vi "test_LogFile Exists on Windows.vi"(8 "error in (no error)":errorcluster, 11 "TestCase in":refnum<class "Telemetry System Tests.lvclass">) -> (0 "error out":errorcluster, 3 "TestCase out":refnum<class "Telemetry System Tests.lvclass">)   [LabVIEW 2019]
uses:
  Telemetry System Tests.lvclass
  e98a7768-7ae7-490c-bb08-fb750c513514.vi
  <vilib>/addons/_JKI Toolkits/VI Tester/TestCase.llb/TestCase.lvclass
  TLCD Test/TLCD Test.lvclass
  C:/Program Files (x86)/National Instruments/LabVIEW 2019/vi.lib/addons/_JKI Toolkits/VI Tester/TestCase.llb/TestCase.lvclass
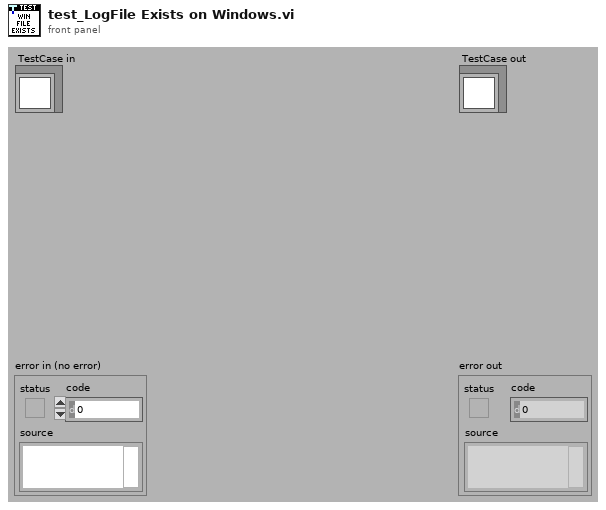
[diagram p1: front panel]
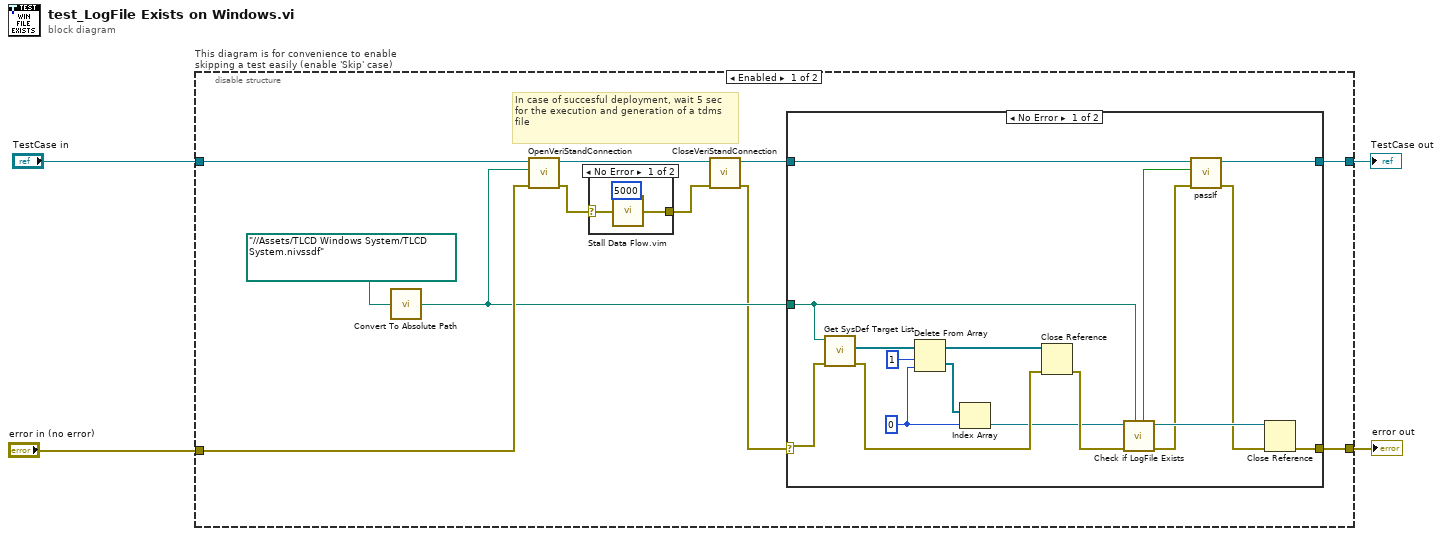
[diagram p0: block diagram]
diagram:
  n1 = disable-structure "This diagram is for convenience to enable skipping a test easily (enable 'Skip' case)" shown="Enabled" {
    disable-tunnel: "TestCase in" -> [w12 w42]
    disable-tunnel: [w14 w40] -> w1
    disable-tunnel: [w15 w41] -> w3
    disable-tunnel: "error in (no error)" -> [w10 w39]
    frame Enabled {
      # "In case of succesful deployment, wait 5 sec for the execution and generation of a tdms file"
      n2 = call "Convert To Absolute Path.vi"("System Definition File Path"=path "../../Assets/TLCD Windows System/TLCD System.nivssdf" ("relative base path")) -> ("Absolute path"=w9:path)
      n3 = call-dynamic "OpenVeriStandConnection.vi"("error in (no error)"=w10, "System Definition File"=w9, "VeriStand Test Case in"=w12) -> ("error out"=w8:errorcluster, "VeriStand Test Case out"=w11:refnum<class "Telemetry System Tests.lvclass">)  [unwired: 6 in, 1 out]
      n4 = case shown="No Error" w8 {
        selector: w8 -> [w37 w38]
        tunnel: [w35 w38] -> w7
        frame No Error {
          n5 = call "Stall Data Flow.vim"("value in"=w37, "milliseconds to wait"=u32 5000) -> ("value out"=w35:errorcluster)  [unwired: 1 out]
        }
        frame Error {
        }
      }
      n6 = call-dynamic "CloseVeriStandConnection.vi"("error in (no error)"=w7, "VeriStand Test Case in"=w11) -> ("error out"=w5:errorcluster, "VeriStand Test Case out"=w6:refnum<class "Telemetry System Tests.lvclass">)  [unwired: 8 in]
      n7 = case shown="No Error" w5 {
        selector: w5 -> [w16 w34]
        tunnel: [w32 w34] -> w15
        tunnel: [w22 w33] -> w14
        tunnel: w9 -> [w18 _]
        tunnel: w6 -> [w17 w33]
        frame No Error {
          w28 = 0 ("index")
          n8 = call "Get SysDef Target List.vi"("error in (no error)"=w16, "System Definition Path"=w18) -> ("error out"=w26:errorcluster, "Target List"=w31:refnum<k24>[])  [unwired: 8 in]
          n9 = Delete From Array(array=w31, length=1, index=w28) -> (deleted portion=w29:refnum<k24>[], array with subset deleted=w27:refnum<k24>[])
          n10 = Index Array(array=w29, index=w28) -> (element=w23:refnum<k24>)
          n11 = Close Reference(reference=w27, error in (no error)=w26) -> (error out=w24:errorcluster)
          n12 = call "Check if LogFile Exists.vi"("System Definition Path"=w18, "error in (no error)"=w24, "Target Refnum in"=w23) -> ("error out"=w20:errorcluster, "Target Refnum out"=w25:refnum<k24>, "LogFile Exists?"=w21:bool)  [unwired: 6 in]
          n13 = call-dynamic "passIf.vi"("error in (no error)"=w20, "pass"=w21, "TestCase in"=w17) -> ("error out"=w19:errorcluster, "TestCase out"=w22:refnum<class "Telemetry System Tests.lvclass">)  [unwired: 7 in]
          n14 = Close Reference(reference=w25, error in (no error)=w19) -> (error out=w32:errorcluster)
        }
        frame Error {
        }
      }
    }
    frame Disabled {
      # "skip test result while test is under development"
      n15 = call <vilib>:"skip.vi"("error in (no error)"=w39, "TestCase in"=w42) -> ("error out"=w41:errorcluster, "TestCase out"=w40:refnum<class "Telemetry System Tests.lvclass">)  [unwired: 8 in]
    }
  }
  "error out" <- w3
  "TestCase out" <- w1
